vi "Envoyer Update Pump.vi"(7 "Message Priority (Normal)":T1=enum."Normal" caption="Priorité des messages (normale)", 8 "error in (no error)":errorcluster caption="entrée d'erreur (pas d'erreur)", 10 "Pump State":bool, 11 "Message Enqueuer":refnum<class "Message Enqueuer.lvclass"> caption="Objet ajoutant des msgs à la file") -> (0 "error out":errorcluster caption="sortie d'erreur", 3 "Message Enqueuer out":refnum<class "Message Enqueuer.lvclass"> caption="Objet ajoutant des msgs à la file en sortie")   [LabVIEW 2015, in "Cooler UI.lvlib" / "Message Update Pump.lvclass"]
doc: "Ce VI envoie le message à un acteur."
uses:
  Message Update Pump.lvclass
  <vilib>/ActorFramework/Message Enqueuer/Message Enqueuer.lvclass
  <vilib>/ActorFramework/Message Enqueuer/Message Priority.ctl
  Message Update Pump.lvclass/Message Update Pump.ctl
  <vilib>/ActorFramework/Message Enqueuer/Message Enqueuer.lvclass/Message Enqueuer.ctl
  <vilib>/ActorFramework/Message Priority Queue/Priority Enqueue.vi
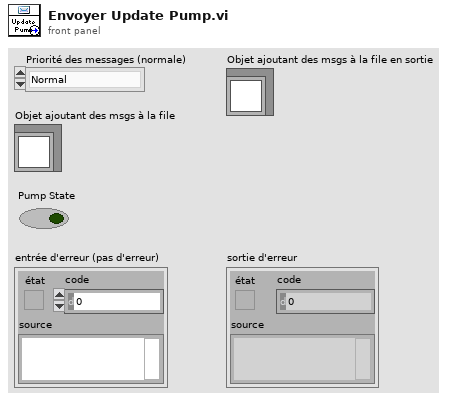
[diagram p1: front panel]
types:
  T1 = typedef "Actor Framework.lvlib/Message Enqueuer.lvclass/Message Priority.ctl" = enum16{"Low", "Normal", "High"}
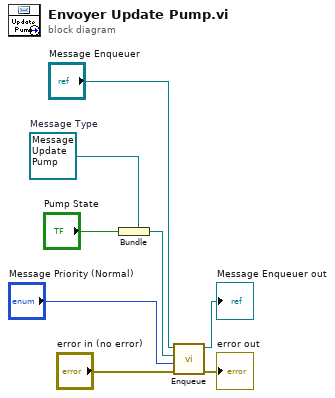
[diagram p0: block diagram]
diagram:
  w5 = refnum<class "Message Update Pump.lvclass"> refnum  # Message Type
  n1 = Bundle(cluster=w5, "Pump State") -> (w4:refnum<class "Message Update Pump.lvclass">)
  n2 = call <vilib>:"Enqueue.vi"("error in (no error)"="error in (no error)", "Message Priority (Normal)"="Message Priority (Normal)", "Message"=w4, "Message Enqueuer in"="Message Enqueuer") -> ("error out"=→"error out":errorcluster, "Message Enqueuer out"=→"Message Enqueuer out":refnum<class "Message Enqueuer.lvclass">)  [unwired: 6 in]
